vi "期末專題TOP.vi"() -> ()   [LabVIEW 2014]
uses:
  <vilib>/Utility/inputDevices.llb/keyboardAcquire.vi
panel:
  out "得分":dbl
  in  "path":path=path "C:/Users/SYUGU/Desktop/期末專題R09522637徐辜建源/期末專題R09522637徐辜建源/期末專題程式/阿一代.wav"
  in  "躲避次數":i32
  out "大便":T1
  in  "大便速度":i32
  out "統神":T2
  out "²Î¯«(ºL":T3
  out "馬路":T4
  # "使用鍵盤的←、→控制統神躲避\n路上的大便，助他度過財務危機"
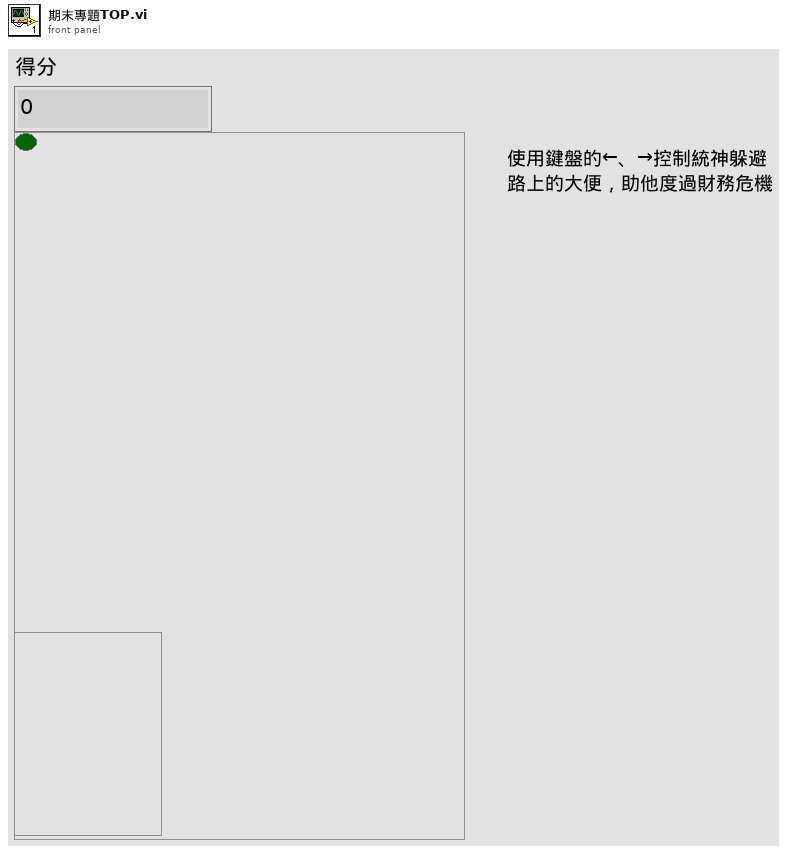
[diagram p1: front panel]
types:
  T1 = typedef "大便.ctl" = bool
  T2 = typedef "統.ctl" = bool
  T3 = typedef "倒下.ctl" = bool
  T4 = typedef "馬路.ctl" = bool
  T5 = enum16{"0", "1", "2", "3", "4", "5", "6", "7", "8", "9", "A", "B", "C", "D", "E", "F", "G", "H", "I", "J", "K", "L", "M", "N", "O", "P", "Q", "R", "S", "T", "U", "V", "W", "X", "Y", "Z", "F1", "F2", "F3", "F4", "F5", "F6", "F7", "F8", "F9", "F10", "F11", "F12", "F13", "F14", "F15", "ADD", "BACK", "BACKSLASH", "CAPITAL", "COMMA", "DECIMAL", "DELETE", "DIVIDE", "DOWN", "END", "EQUALS", "ESCAPE", "GRAVE (`)", "HOME", "INSERT", "LBRACKET", "LCONTROL", "LEFT", "L ALT", "LSHIFT", "LWIN", "MINUS", "MULTIPLY", "NEXT", "NUMLOCK", "NUMPAD_0", "NUMPAD_1", "NUMPAD_2", "NUMPAD_3", "NUMPAD_4", "NUMPAD_5", "NUMPAD_6", "NUMPAD_7", "NUMPAD_8", "NUMPAD_9", "PAUSE", "PERIOD", "PRIOR (PG UP)", "RBRACKET", "RCONTROL", "RETURN", "RIGHT", "R ALT", "RSHIFT", "RWIN", "SCROLL", "SEMICOLON", "SLASH", "SPACE", "SUBTRACT", "TAB", "UP", "ENTER (num pad)", "' (quote)"}[]
  T6 = cluster{"keys pressed[0]":enum16{"0", "1", "2", "3", "4", "5", "6", "7", "8", "9", "A", "B", "C", "D", "E", "F", "G", "H", "I", "J", "K", "L", "M", "N", "O", "P", "Q", "R", "S", "T", "U", "V", "W", "X", "Y", "Z", "F1", "F2", "F3", "F4", "F5", "F6", "F7", "F8", "F9", "F10", "F11", "F12", "F13", "F14", "F15", "ADD", "BACK", "BACKSLASH", "CAPITAL", "COMMA", "DECIMAL", "DELETE", "DIVIDE", "DOWN", "END", "EQUALS", "ESCAPE", "GRAVE (`)", "HOME", "INSERT", "LBRACKET", "LCONTROL", "LEFT", "L ALT", "LSHIFT", "LWIN", "MINUS", "MULTIPLY", "NEXT", "NUMLOCK", "NUMPAD_0", "NUMPAD_1", "NUMPAD_2", "NUMPAD_3", "NUMPAD_4", "NUMPAD_5", "NUMPAD_6", "NUMPAD_7", "NUMPAD_8", "NUMPAD_9", "PAUSE", "PERIOD", "PRIOR (PG UP)", "RBRACKET", "RCONTROL", "RETURN", "RIGHT", "R ALT", "RSHIFT", "RWIN", "SCROLL", "SEMICOLON", "SLASH", "SPACE", "SUBTRACT", "TAB", "UP", "ENTER (num pad)", "' (quote)"}, "keys pressed[1]":enum16{"0", "1", "2", "3", "4", "5", "6", "7", "8", "9", "A", "B", "C", "D", "E", "F", "G", "H", "I", "J", "K", "L", "M", "N", "O", "P", "Q", "R", "S", "T", "U", "V", "W", "X", "Y", "Z", "F1", "F2", "F3", "F4", "F5", "F6", "F7", "F8", "F9", "F10", "F11", "F12", "F13", "F14", "F15", "ADD", "BACK", "BACKSLASH", "CAPITAL", "COMMA", "DECIMAL", "DELETE", "DIVIDE", "DOWN", "END", "EQUALS", "ESCAPE", "GRAVE (`)", "HOME", "INSERT", "LBRACKET", "LCONTROL", "LEFT", "L ALT", "LSHIFT", "LWIN", "MINUS", "MULTIPLY", "NEXT", "NUMLOCK", "NUMPAD_0", "NUMPAD_1", "NUMPAD_2", "NUMPAD_3", "NUMPAD_4", "NUMPAD_5", "NUMPAD_6", "NUMPAD_7", "NUMPAD_8", "NUMPAD_9", "PAUSE", "PERIOD", "PRIOR (PG UP)", "RBRACKET", "RCONTROL", "RETURN", "RIGHT", "R ALT", "RSHIFT", "RWIN", "SCROLL", "SEMICOLON", "SLASH", "SPACE", "SUBTRACT", "TAB", "UP", "ENTER (num pad)", "' (quote)"}, "keys pressed[2]":enum16{"0", "1", "2", "3", "4", "5", "6", "7", "8", "9", "A", "B", "C", "D", "E", "F", "G", "H", "I", "J", "K", "L", "M", "N", "O", "P", "Q", "R", "S", "T", "U", "V", "W", "X", "Y", "Z", "F1", "F2", "F3", "F4", "F5", "F6", "F7", "F8", "F9", "F10", "F11", "F12", "F13", "F14", "F15", "ADD", "BACK", "BACKSLASH", "CAPITAL", "COMMA", "DECIMAL", "DELETE", "DIVIDE", "DOWN", "END", "EQUALS", "ESCAPE", "GRAVE (`)", "HOME", "INSERT", "LBRACKET", "LCONTROL", "LEFT", "L ALT", "LSHIFT", "LWIN", "MINUS", "MULTIPLY", "NEXT", "NUMLOCK", "NUMPAD_0", "NUMPAD_1", "NUMPAD_2", "NUMPAD_3", "NUMPAD_4", "NUMPAD_5", "NUMPAD_6", "NUMPAD_7", "NUMPAD_8", "NUMPAD_9", "PAUSE", "PERIOD", "PRIOR (PG UP)", "RBRACKET", "RCONTROL", "RETURN", "RIGHT", "R ALT", "RSHIFT", "RWIN", "SCROLL", "SEMICOLON", "SLASH", "SPACE", "SUBTRACT", "TAB", "UP", "ENTER (num pad)", "' (quote)"}, "keys pressed[3]":enum16{"0", "1", "2", "3", "4", "5", "6", "7", "8", "9", "A", "B", "C", "D", "E", "F", "G", "H", "I", "J", "K", "L", "M", "N", "O", "P", "Q", "R", "S", "T", "U", "V", "W", "X", "Y", "Z", "F1", "F2", "F3", "F4", "F5", "F6", "F7", "F8", "F9", "F10", "F11", "F12", "F13", "F14", "F15", "ADD", "BACK", "BACKSLASH", "CAPITAL", "COMMA", "DECIMAL", "DELETE", "DIVIDE", "DOWN", "END", "EQUALS", "ESCAPE", "GRAVE (`)", "HOME", "INSERT", "LBRACKET", "LCONTROL", "LEFT", "L ALT", "LSHIFT", "LWIN", "MINUS", "MULTIPLY", "NEXT", "NUMLOCK", "NUMPAD_0", "NUMPAD_1", "NUMPAD_2", "NUMPAD_3", "NUMPAD_4", "NUMPAD_5", "NUMPAD_6", "NUMPAD_7", "NUMPAD_8", "NUMPAD_9", "PAUSE", "PERIOD", "PRIOR (PG UP)", "RBRACKET", "RCONTROL", "RETURN", "RIGHT", "R ALT", "RSHIFT", "RWIN", "SCROLL", "SEMICOLON", "SLASH", "SPACE", "SUBTRACT", "TAB", "UP", "ENTER (num pad)", "' (quote)"}, "keys pressed[4]":enum16{"0", "1", "2", "3", "4", "5", "6", "7", "8", "9", "A", "B", "C", "D", "E", "F", "G", "H", "I", "J", "K", "L", "M", "N", "O", "P", "Q", "R", "S", "T", "U", "V", "W", "X", "Y", "Z", "F1", "F2", "F3", "F4", "F5", "F6", "F7", "F8", "F9", "F10", "F11", "F12", "F13", "F14", "F15", "ADD", "BACK", "BACKSLASH", "CAPITAL", "COMMA", "DECIMAL", "DELETE", "DIVIDE", "DOWN", "END", "EQUALS", "ESCAPE", "GRAVE (`)", "HOME", "INSERT", "LBRACKET", "LCONTROL", "LEFT", "L ALT", "LSHIFT", "LWIN", "MINUS", "MULTIPLY", "NEXT", "NUMLOCK", "NUMPAD_0", "NUMPAD_1", "NUMPAD_2", "NUMPAD_3", "NUMPAD_4", "NUMPAD_5", "NUMPAD_6", "NUMPAD_7", "NUMPAD_8", "NUMPAD_9", "PAUSE", "PERIOD", "PRIOR (PG UP)", "RBRACKET", "RCONTROL", "RETURN", "RIGHT", "R ALT", "RSHIFT", "RWIN", "SCROLL", "SEMICOLON", "SLASH", "SPACE", "SUBTRACT", "TAB", "UP", "ENTER (num pad)", "' (quote)"}, "keys pressed[5]":enum16{"0", "1", "2", "3", "4", "5", "6", "7", "8", "9", "A", "B", "C", "D", "E", "F", "G", "H", "I", "J", "K", "L", "M", "N", "O", "P", "Q", "R", "S", "T", "U", "V", "W", "X", "Y", "Z", "F1", "F2", "F3", "F4", "F5", "F6", "F7", "F8", "F9", "F10", "F11", "F12", "F13", "F14", "F15", "ADD", "BACK", "BACKSLASH", "CAPITAL", "COMMA", "DECIMAL", "DELETE", "DIVIDE", "DOWN", "END", "EQUALS", "ESCAPE", "GRAVE (`)", "HOME", "INSERT", "LBRACKET", "LCONTROL", "LEFT", "L ALT", "LSHIFT", "LWIN", "MINUS", "MULTIPLY", "NEXT", "NUMLOCK", "NUMPAD_0", "NUMPAD_1", "NUMPAD_2", "NUMPAD_3", "NUMPAD_4", "NUMPAD_5", "NUMPAD_6", "NUMPAD_7", "NUMPAD_8", "NUMPAD_9", "PAUSE", "PERIOD", "PRIOR (PG UP)", "RBRACKET", "RCONTROL", "RETURN", "RIGHT", "R ALT", "RSHIFT", "RWIN", "SCROLL", "SEMICOLON", "SLASH", "SPACE", "SUBTRACT", "TAB", "UP", "ENTER (num pad)", "' (quote)"}, "keys pressed[6]":enum16{"0", "1", "2", "3", "4", "5", "6", "7", "8", "9", "A", "B", "C", "D", "E", "F", "G", "H", "I", "J", "K", "L", "M", "N", "O", "P", "Q", "R", "S", "T", "U", "V", "W", "X", "Y", "Z", "F1", "F2", "F3", "F4", "F5", "F6", "F7", "F8", "F9", "F10", "F11", "F12", "F13", "F14", "F15", "ADD", "BACK", "BACKSLASH", "CAPITAL", "COMMA", "DECIMAL", "DELETE", "DIVIDE", "DOWN", "END", "EQUALS", "ESCAPE", "GRAVE (`)", "HOME", "INSERT", "LBRACKET", "LCONTROL", "LEFT", "L ALT", "LSHIFT", "LWIN", "MINUS", "MULTIPLY", "NEXT", "NUMLOCK", "NUMPAD_0", "NUMPAD_1", "NUMPAD_2", "NUMPAD_3", "NUMPAD_4", "NUMPAD_5", "NUMPAD_6", "NUMPAD_7", "NUMPAD_8", "NUMPAD_9", "PAUSE", "PERIOD", "PRIOR (PG UP)", "RBRACKET", "RCONTROL", "RETURN", "RIGHT", "R ALT", "RSHIFT", "RWIN", "SCROLL", "SEMICOLON", "SLASH", "SPACE", "SUBTRACT", "TAB", "UP", "ENTER (num pad)", "' (quote)"}, "keys pressed[7]":enum16{"0", "1", "2", "3", "4", "5", "6", "7", "8", "9", "A", "B", "C", "D", "E", "F", "G", "H", "I", "J", "K", "L", "M", "N", "O", "P", "Q", "R", "S", "T", "U", "V", "W", "X", "Y", "Z", "F1", "F2", "F3", "F4", "F5", "F6", "F7", "F8", "F9", "F10", "F11", "F12", "F13", "F14", "F15", "ADD", "BACK", "BACKSLASH", "CAPITAL", "COMMA", "DECIMAL", "DELETE", "DIVIDE", "DOWN", "END", "EQUALS", "ESCAPE", "GRAVE (`)", "HOME", "INSERT", "LBRACKET", "LCONTROL", "LEFT", "L ALT", "LSHIFT", "LWIN", "MINUS", "MULTIPLY", "NEXT", "NUMLOCK", "NUMPAD_0", "NUMPAD_1", "NUMPAD_2", "NUMPAD_3", "NUMPAD_4", "NUMPAD_5", "NUMPAD_6", "NUMPAD_7", "NUMPAD_8", "NUMPAD_9", "PAUSE", "PERIOD", "PRIOR (PG UP)", "RBRACKET", "RCONTROL", "RETURN", "RIGHT", "R ALT", "RSHIFT", "RWIN", "SCROLL", "SEMICOLON", "SLASH", "SPACE", "SUBTRACT", "TAB", "UP", "ENTER (num pad)", "' (quote)"}, "keys pressed[8]":enum16{"0", "1", "2", "3", "4", "5", "6", "7", "8", "9", "A", "B", "C", "D", "E", "F", "G", "H", "I", "J", "K", "L", "M", "N", "O", "P", "Q", "R", "S", "T", "U", "V", "W", "X", "Y", "Z", "F1", "F2", "F3", "F4", "F5", "F6", "F7", "F8", "F9", "F10", "F11", "F12", "F13", "F14", "F15", "ADD", "BACK", "BACKSLASH", "CAPITAL", "COMMA", "DECIMAL", "DELETE", "DIVIDE", "DOWN", "END", "EQUALS", "ESCAPE", "GRAVE (`)", "HOME", "INSERT", "LBRACKET", "LCONTROL", "LEFT", "L ALT", "LSHIFT", "LWIN", "MINUS", "MULTIPLY", "NEXT", "NUMLOCK", "NUMPAD_0", "NUMPAD_1", "NUMPAD_2", "NUMPAD_3", "NUMPAD_4", "NUMPAD_5", "NUMPAD_6", "NUMPAD_7", "NUMPAD_8", "NUMPAD_9", "PAUSE", "PERIOD", "PRIOR (PG UP)", "RBRACKET", "RCONTROL", "RETURN", "RIGHT", "R ALT", "RSHIFT", "RWIN", "SCROLL", "SEMICOLON", "SLASH", "SPACE", "SUBTRACT", "TAB", "UP", "ENTER (num pad)", "' (quote)"}}
  T7 = enum16{"0", "1", "2", "3", "4", "5", "6", "7", "8", "9", "A", "B", "C", "D", "E", "F", "G", "H", "I", "J", "K", "L", "M", "N", "O", "P", "Q", "R", "S", "T", "U", "V", "W", "X", "Y", "Z", "F1", "F2", "F3", "F4", "F5", "F6", "F7", "F8", "F9", "F10", "F11", "F12", "F13", "F14", "F15", "ADD", "BACK", "BACKSLASH", "CAPITAL", "COMMA", "DECIMAL", "DELETE", "DIVIDE", "DOWN", "END", "EQUALS", "ESCAPE", "GRAVE (`)", "HOME", "INSERT", "LBRACKET", "LCONTROL", "LEFT", "L ALT", "LSHIFT", "LWIN", "MINUS", "MULTIPLY", "NEXT", "NUMLOCK", "NUMPAD_0", "NUMPAD_1", "NUMPAD_2", "NUMPAD_3", "NUMPAD_4", "NUMPAD_5", "NUMPAD_6", "NUMPAD_7", "NUMPAD_8", "NUMPAD_9", "PAUSE", "PERIOD", "PRIOR (PG UP)", "RBRACKET", "RCONTROL", "RETURN", "RIGHT", "R ALT", "RSHIFT", "RWIN", "SCROLL", "SEMICOLON", "SLASH", "SPACE", "SUBTRACT", "TAB", "UP", "ENTER (num pad)", "' (quote)"}
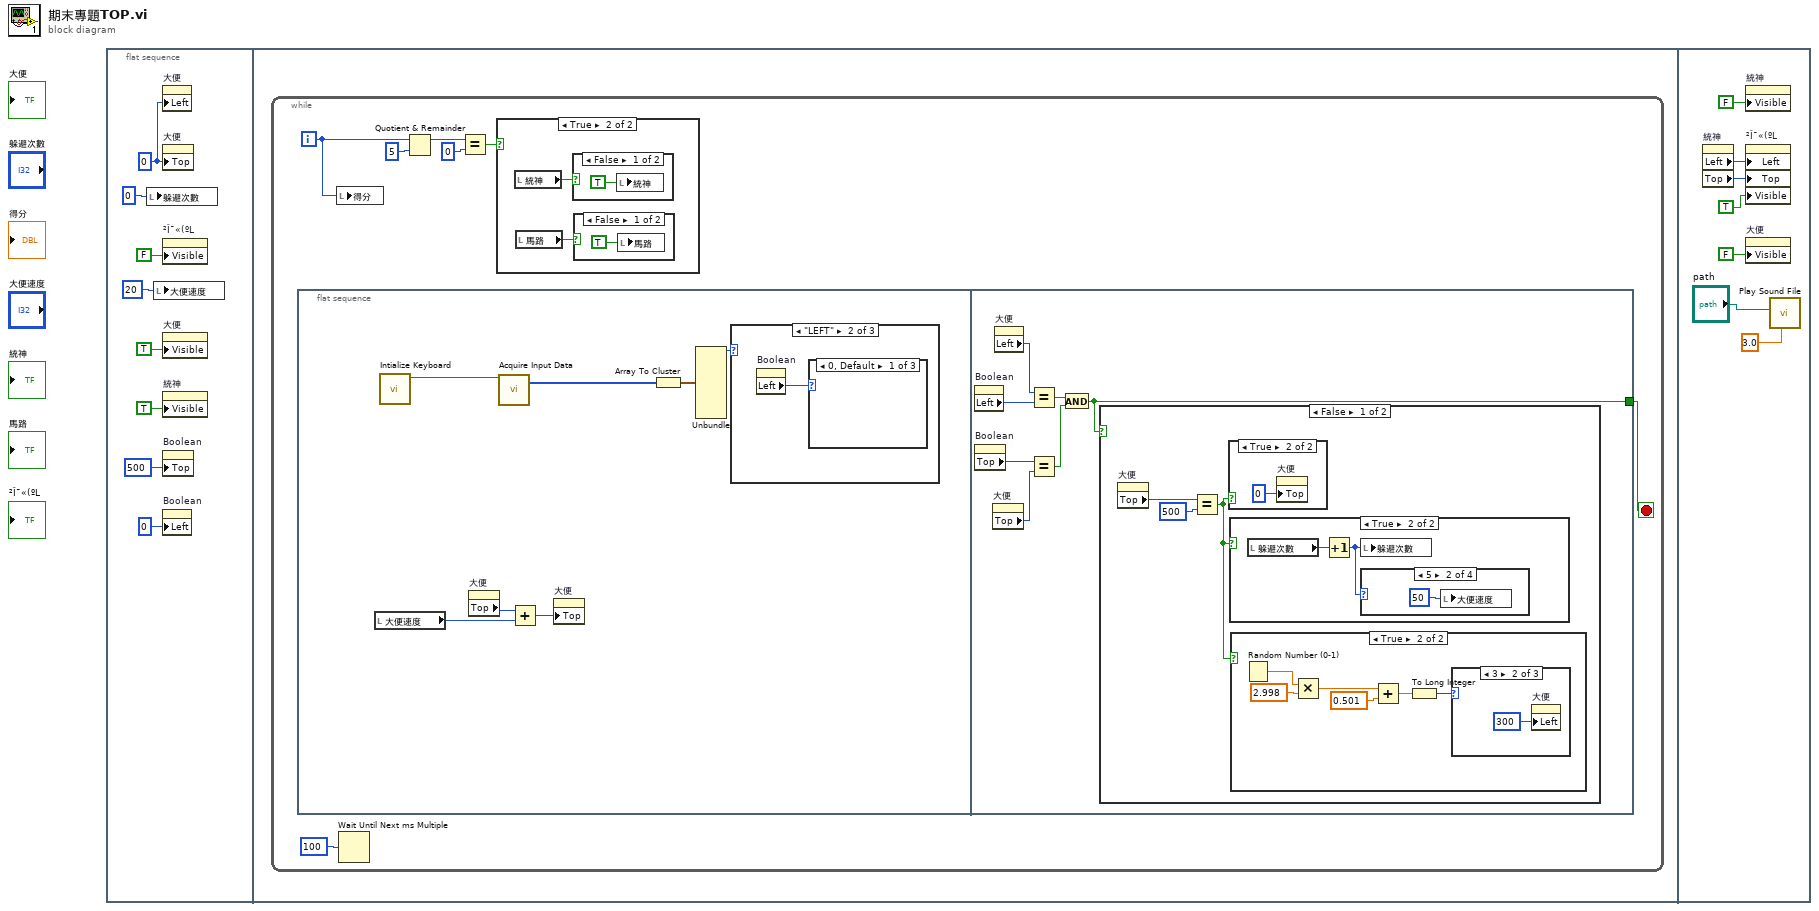
[diagram p0: block diagram]
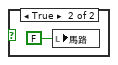
[diagram p3: hidden frame]
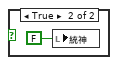
[diagram p4: hidden frame]
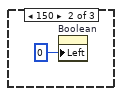
[diagram p6: hidden frame]
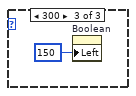
[diagram p7: hidden frame]
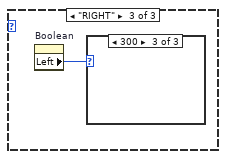
[diagram p8: hidden frame]
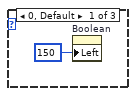
[diagram p9: hidden frame]
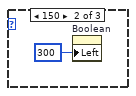
[diagram p10: hidden frame]
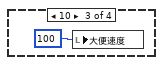
[diagram p13: hidden frame]
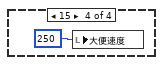
[diagram p14: hidden frame]
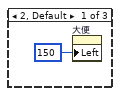
[diagram p16: hidden frame]
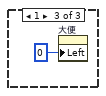
[diagram p17: hidden frame]
diagram:
  n1 = flat-sequence {
    frame #0 {
      w8 = 0
      n2 = local write "躲避次數"(0 ("躲避次數")) -> ()
      n3 = local write "大便速度"(20 ("大便速度")) -> ()
      n4 = property on="大便" class="Bool (strict)"("Left"=w8) -> ()  [unwired: 2 in, 2 out]
      n5 = property on="大便" class="Bool (strict)"("Top"=w8) -> ()  [unwired: 2 in, 2 out]
      n6 = property on="²Î¯«(ºL" class="Bool (strict)"("Visible"=FALSE) -> ()  [unwired: 2 in, 2 out]
      n7 = property on="大便" class="Bool (strict)"("Visible"=TRUE) -> ()  [unwired: 2 in, 2 out]
      n8 = property on="統神" class="Bool (strict)"("Visible"=TRUE) -> ()  [unwired: 2 in, 2 out]
      n9 = property on="Boolean" class="Bool (strict)"("Top"=500 ("Position:Top")) -> ()  [unwired: 2 in, 2 out]
      n10 = property on="Boolean" class="Bool (strict)"("Left"=0 ("Position:Left")) -> ()  [unwired: 2 in, 2 out]
    }
    frame #1 {
      n11 = while {
        i -> [w9]
        stop <- w14 stop-if-true
        n12 = flat-sequence {
          tunnel: [w35] -> w14
          frame #0 {
            n13 = local read "大便速度"() -> (w22:i32)
            n14 = call <vilib>:"Intialize Keyboard.vi"() -> ("device ID"=w26:refnum<k1>)  [unwired: 10 in, 1 out]
            n15 = property on="大便" class="Bool (strict)"() -> ("Top"=w28:i32)  [unwired: 2 in, 2 out]
            n16 = call-poly <vilib>:"Acquire Input Data.vi"("device ID"=w26) -> ("keys pressed"=w23:T5)  [unwired: 16 in, 2 out]
            n17 = Add(x=w28, y=w22) -> (x+y=w27:i32)
            n18 = property on="大便" class="Bool (strict)"("Top"=w27) -> ()  [unwired: 2 in, 2 out]
            n19 = Array To Cluster(array=w23) -> (cluster=w24:T6)
            n20 = Unbundle(w24) -> ("keys pressed[0]"=w25:T7)  [unwired: 8 out]
            n21 = case shown="\"LEFT\"" w25 {
              frame "0", Default {
              }
              frame "LEFT" {
                n22 = property on="Boolean" class="Bool (strict)"() -> ("Left"=w29:i32)  [unwired: 2 in, 2 out]
                n23 = case shown="0, Default" w29 {
                  frame 0, Default {
                  }
                  frame 150 {
                    n24 = property on="Boolean" class="Bool (strict)"("Left"=0 ("Position:Left")) -> ()  [unwired: 2 in, 2 out]
                  }
                  frame 300 {
                    n25 = property on="Boolean" class="Bool (strict)"("Left"=150 ("Position:Left")) -> ()  [unwired: 2 in, 2 out]
                  }
                }
              }
              frame "RIGHT" {
                n26 = property on="Boolean" class="Bool (strict)"() -> ("Left"=w32:i32)  [unwired: 2 in, 2 out]
                n27 = case shown="300" w32 {
                  frame 0, Default {
                    n28 = property on="Boolean" class="Bool (strict)"("Left"=150) -> ()  [unwired: 2 in, 2 out]
                  }
                  frame 150 {
                    n29 = property on="Boolean" class="Bool (strict)"("Left"=300 ("Position:Left")) -> ()  [unwired: 2 in, 2 out]
                  }
                  frame 300 {
                  }
                }
              }
            }
          }
          frame #1 {
            n30 = property on="Boolean" class="Bool (strict)"() -> ("Left"=w37:i32)  [unwired: 2 in, 2 out]
            n31 = property on="Boolean" class="Bool (strict)"() -> ("Top"=w38:i32)  [unwired: 2 in, 2 out]
            n32 = property on="大便" class="Bool (strict)"() -> ("Top"=w39:i32)  [unwired: 2 in, 2 out]
            n33 = property on="大便" class="Bool (strict)"() -> ("Left"=w36:i32)  [unwired: 2 in, 2 out]
            n34 = Equal?(x=w36, y=w37) -> (x = y?=w40:bool)
            n35 = Equal?(x=w38, y=w39) -> (x = y?=w41:bool)
            n36 = And(x=w40, y=w41) -> (x .and. y?=w35:bool)
            n37 = case shown="False" w35 {
              frame False {
                n38 = property on="大便" class="Bool (strict)"() -> ("Top"=w44:i32)  [unwired: 2 in, 2 out]
                n39 = Equal?(x=w44, y=500) -> (x = y?=w42:bool)
                n40 = case shown="True" w42 {
                  frame False {
                  }
                  frame True {
                    n41 = property on="大便" class="Bool (strict)"("Top"=0) -> ()  [unwired: 2 in, 2 out]
                  }
                }
                n42 = case shown="True" w42 {
                  frame False {
                  }
                  frame True {
                    n43 = local read "躲避次數"() -> (w46:i32)
                    n44 = Increment(x=w46) -> (x+1=w45:i32)
                    n45 = local write "躲避次數"(w45) -> ()
                    n46 = case shown="5" w45 {
                      frame 0, Default {
                      }
                      frame 5 {
                        n47 = local write "大便速度"(50 ("大便速度")) -> ()
                      }
                      frame 10 {
                        n48 = local write "大便速度"(100 ("大便速度")) -> ()
                      }
                      frame 15 {
                        n49 = local write "大便速度"(250 ("大便速度")) -> ()
                      }
                    }
                  }
                }
                n50 = case shown="True" w42 {
                  frame False {
                  }
                  frame True {
                    n51 = Random Number (0-1)() -> (number: 0 to 1=w55:dbl)
                    n52 = Multiply(x=w55, y=2.998) -> (x*y=w53:dbl)
                    n53 = Add(x=w53, y=0.501) -> (x+y=w51:dbl)
                    n54 = To Long Integer(number=w51) -> (32bit integer=w50:i32)
                    n55 = case shown="3" w50 {
                      frame 2, Default {
                        n56 = property on="大便" class="Bool (strict)"("Left"=150) -> ()  [unwired: 2 in, 2 out]
                      }
                      frame 3 {
                        n57 = property on="大便" class="Bool (strict)"("Left"=300) -> ()  [unwired: 2 in, 2 out]
                      }
                      frame 1 {
                        n58 = property on="大便" class="Bool (strict)"("Left"=0) -> ()  [unwired: 2 in, 2 out]
                      }
                    }
                  }
                }
              }
              frame True {
              }
            }
          }
        }
        n59 = local write "得分"(w9) -> ()
        n60 = Wait Until Next ms Multiple(millisecond multiple=u32 100) -> ()  [unwired: 1 out]
        n61 = Quotient & Remainder(x=w9, y=5) -> (x-y*floor(x/y)=w12:i32)  [unwired: 1 out]
        n62 = Equal?(x=w12, y=0) -> (x = y?=w10:bool)
        n63 = case shown="True" w10 {
          frame False {
          }
          frame True {
            n64 = local read "統神"() -> (w17:T2)
            n65 = local read "馬路"() -> (w16:T4)
            n66 = case shown="False" w17 {
              frame False {
                n67 = local write "統神"(TRUE) -> ()
              }
              frame True {
                n68 = local write "統神"(FALSE) -> ()
              }
            }
            n69 = case shown="False" w16 {
              frame False {
                n70 = local write "馬路"(T4 TRUE ("馬路")) -> ()
              }
              frame True {
                n71 = local write "馬路"(T4 FALSE ("馬路")) -> ()
              }
            }
          }
        }
      }
    }
    frame #2 {
      n72 = property on="統神" class="Bool (strict)"() -> ("Left"=w66:i32, "Top"=w65:i32)  [unwired: 2 in, 2 out]
      n73 = property on="統神" class="Bool (strict)"("Visible"=FALSE) -> ()  [unwired: 2 in, 2 out]
      n74 = property on="²Î¯«(ºL" class="Bool (strict)"("Left"=w66, "Top"=w65, "Visible"=TRUE ("Blinking")) -> ()  [unwired: 2 in, 2 out]
      n75 = property on="大便" class="Bool (strict)"("Visible"=FALSE) -> ()  [unwired: 2 in, 2 out]
      n76 = call <vilib>:"Play Sound File.vi"("timeout (sec)"=3.0, "path"="path") -> ()  [unwired: 8 in, 2 out]
    }
  }
